vi "Stop watch.vi"(7 "Time to wait, mS":dbl format="%#_13g", 13 "reset timer":bool) -> (2 "Elapsed time, ms":u32, 8 "Timer up":bool)   [LabVIEW 2014, in "Stop watch.lvlib"]
uses:
  Stop watch.lvlib
panel:
  out "last time":u32
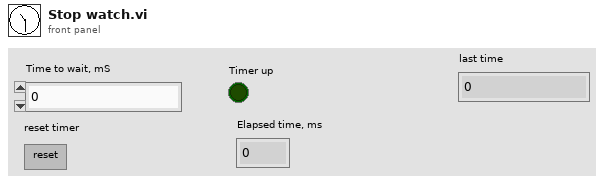
[diagram p1: front panel]
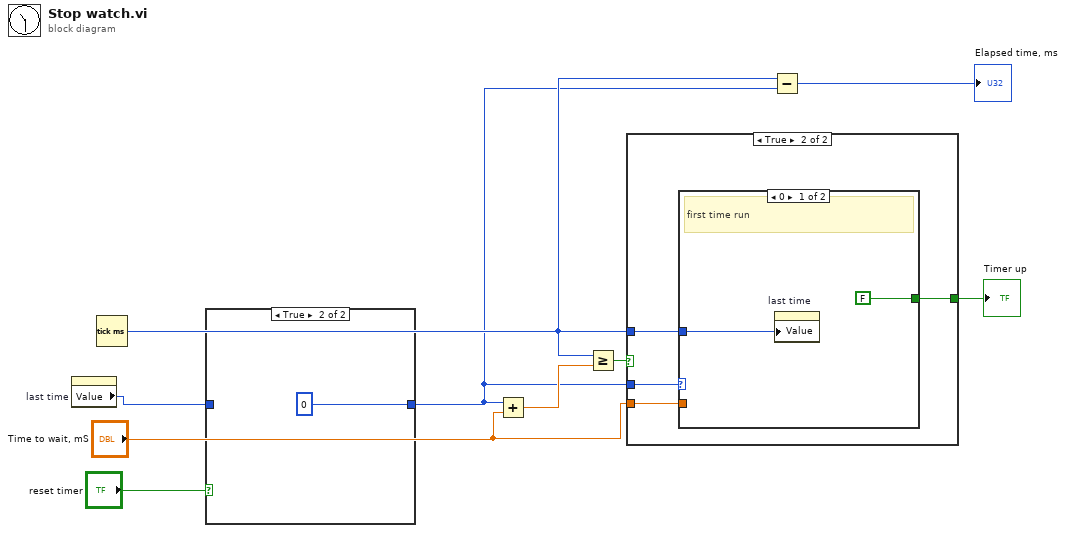
[diagram p0: block diagram]
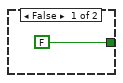
[diagram p3: hidden frame]
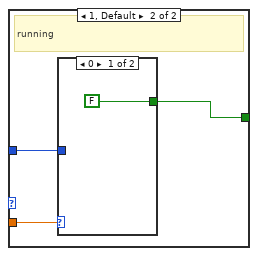
[diagram p4: hidden frame]
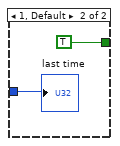
[diagram p5: hidden frame]
diagram:
  n1 = property on="last time" class="DigNum (strict)"() -> ("Value"=w2:u32)  [unwired: 2 in, 2 out]
  n2 = Tick Count (ms)() -> (millisecond timer value=w6:u32)
  n3 = case shown="True" "reset timer" {
    tunnel: w2 -> [w10 _]
    tunnel: [w10 u32 0 ("last time")] -> w1
    frame False {
    }
    frame True {
    }
  }
  n4 = Add(x=w1, y="Time to wait, mS") -> (x+y=w9:dbl)
  n5 = Greater Or Equal?(x=w6, y=w9) -> (x >= y?=w8:bool)
  n6 = case shown="True" w8 {
    tunnel: [FALSE w16] -> w7
    tunnel: w6 -> [_ w15]
    tunnel: w1 -> [_ w14]
    tunnel: "Time to wait, mS" -> [_ w13]
    frame False {
    }
    frame True {
      n7 = case shown="0" w14 {
        tunnel: [FALSE w21] -> w16
        tunnel: w15 -> [w17 w20]
        tunnel: w13 -> [_ w19]
        frame 0 {
          # "first time run"
          n8 = property on="last time" class="DigNum (strict)"("Value"=w17) -> ()  [unwired: 2 in, 2 out]
        }
        frame 1, Default {
          # "running"
          n9 = case shown="0" w19 {
            tunnel: [FALSE TRUE] -> w21
            tunnel: w20 -> [_ w23]
            frame 0 {
            }
            frame 1, Default {
              "last time" <- w23
            }
          }
        }
      }
    }
  }
  "Timer up" <- w7
  n10 = Subtract(x=w6, y=w1) -> (x-y=→"Elapsed time, ms":u32)
